vi "New OR Replicate (SubVI).vi"(0 "PASS OR FAIL Pulse":bool, 2 "Replicate Button":bool, 3 "New Button":bool, 5 "New Case Signal":bool) -> (16 "Case Output":T1(ring), 17 "PASS OR FAIL Latch":bool, 18 "Replicate Signal":bool, 19 "Next Case Signal":bool)   [LabVIEW 2009]
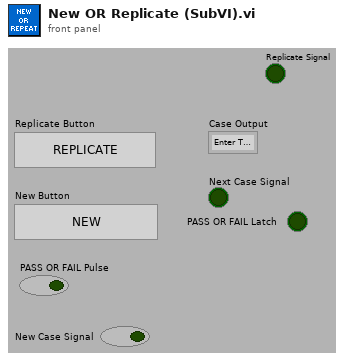
[diagram p1: front panel]
types:
  T1 = enum16{"Enter Test Details", "Warm-Up Cycles", "Test Mode", "Evaluate & Save"}
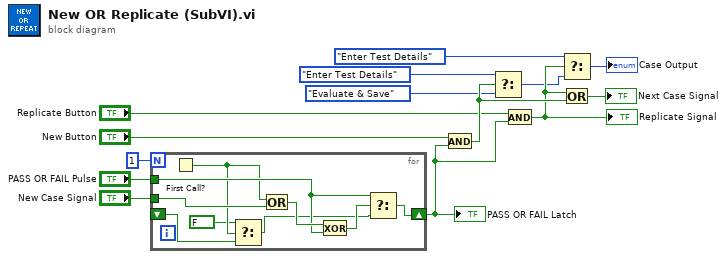
[diagram p0: block diagram]
diagram:
  n1 = for {
    N: 1 -> [_]
    shift-right: [w22] -> w6
    shift-left: _ -> [w16]
    tunnel: "New Case Signal" -> [w19]
    tunnel: "PASS OR FAIL Pulse" -> [w20]
    n2 = First Call?() -> (First Call?: T/F=w18:bool)
    n3 = Select(t=FALSE ("x .and. y?"), s=w18, f=w16) -> (s? t:f=w15:bool)
    n4 = Or(x=w18, y=w19) -> (x .or. y?=w21:bool)
    n5 = Exclusive Or(1:w20, 2:w21) -> (0:w23:bool)
    n6 = Select(t=w20, s=w23, f=w15) -> (s? t:f=w22:bool)
  }
  "PASS OR FAIL Latch" <- w6
  n7 = And(x="New Button", y=w6) -> (x .and. y?=w13:bool)
  n8 = Select(t=T1."Enter Test Details" ("Start Case"), s=w13, f=T1."Evaluate & Save") -> (s? t:f=w10:T1)
  n9 = And(x="Replicate Button", y=w6) -> (x .and. y?=w12:bool)
  "Replicate Signal" <- w12
  n10 = Select(t=T1."Enter Test Details" ("Start Case"), s=w12, f=w10) -> (s? t:f=→"Case Output":T1)
  n11 = Or(x=w12, y=w13) -> (x .or. y?=→"Next Case Signal":bool)
